vi "CursorGet.vi"(8 "错误输入":errorcluster caption="错误输入（无错误）", 11 "WG":refnum<vi>) -> (0 "错误输出":errorcluster, 2 "MIN":dbl, 3 "MAX":dbl)   [LabVIEW 2012]
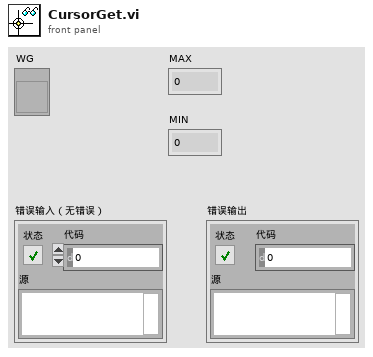
[diagram p1: front panel]
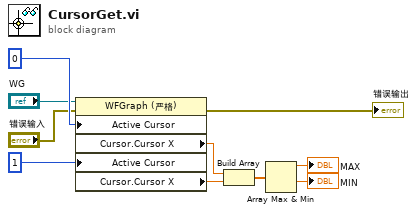
[diagram p0: block diagram]
diagram:
  n1 = property on="属性节点" class="WFGraph (严格)"(reference="WG", error in="错误输入", "Active Cursor"=u32 0 ("活动游标"), "Active Cursor"=u32 1 ("活动游标")) -> (error out=→"错误输出":errorcluster, "Cursor.Cursor X"=w4:dbl, "Cursor.Cursor X"=w5:dbl)  [unwired: 1 out]
  n2 = Build Array(w4, w5) -> (w6:dbl[])
  n3 = Array Max & Min(array=w6) -> (max value=→"MAX":dbl, min value=→"MIN":dbl)  [unwired: 2 out]
